vi "Cooler OFF.vi"(8 "error in (no error)":errorcluster, 11 "Cooler in":refnum<class "Simulated_Cooler.lvclass">) -> (0 "error out":errorcluster, 3 "Cooler out":refnum<class "Simulated_Cooler.lvclass">)   [LabVIEW 2018, in "Simulated_Cooler.lvclass"]
uses:
  Simulated_Cooler.lvclass
  Simulated_Cooler.lvclass/Simulated_Cooler.ctl
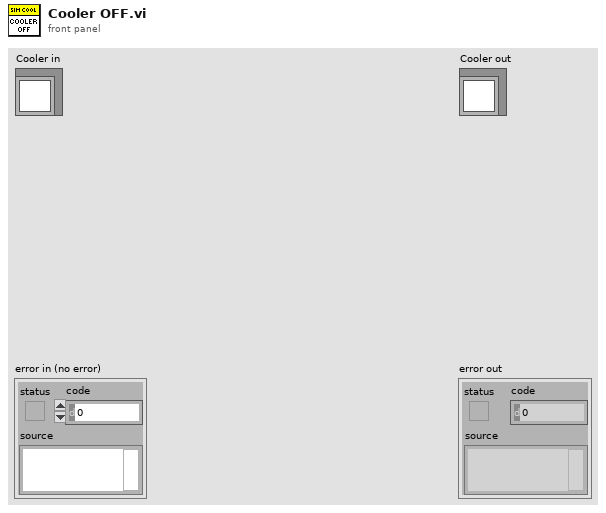
[diagram p1: front panel]
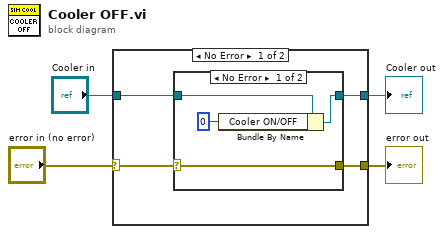
[diagram p0: block diagram]
diagram:
  n1 = case shown="No Error" "error in (no error)" {
    selector: "error in (no error)" -> [w5 w16]
    tunnel: [w8 w16] -> w2
    tunnel: [w6 w15] -> w3
    tunnel: "Cooler in" -> [w7 w15]
    frame No Error {
      n2 = case shown="No Error" w5 {
        selector: w5 -> [w12 w13]
        tunnel: [w12 w13] -> w8
        tunnel: w7 -> [w11 w14]
        tunnel: [w10 w14] -> w6
        frame No Error {
          n3 = Bundle By Name(cluster=w11, "Cooler ON/OFF"=u8 0) -> (w10:refnum<class "Simulated_Cooler.lvclass">)
        }
        frame Error {
        }
      }
    }
    frame Error {
    }
  }
  "error out" <- w2
  "Cooler out" <- w3
